vi "ESC controller 180319.vi"() -> ()   [LabVIEW 2022 SP3]
uses:
  <vilib>/Instr/_visa.llb/VISA Configure Serial Port (Instr).vi
panel:
  in  "OK Button":bool
  in  "Motor Capacity %":dbl(slide) scale=0.0..100.0
  in  "VISA resource name":refnum<visa-resource-name>="COM37"
  in  "exit":bool
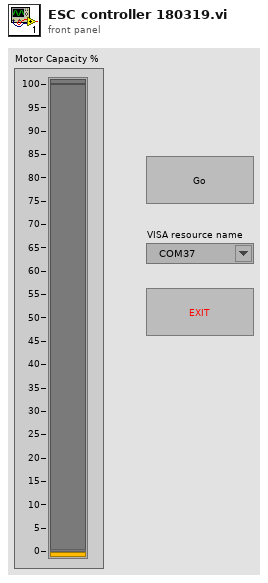
[diagram p1: front panel]
types:
  T1 = cluster{"baud rate":u32, "data bits":u16, "parity":enum16{"None", "Odd", "Even", "Mark", "Space"}, "stop bits":u16, "flow control":u16}
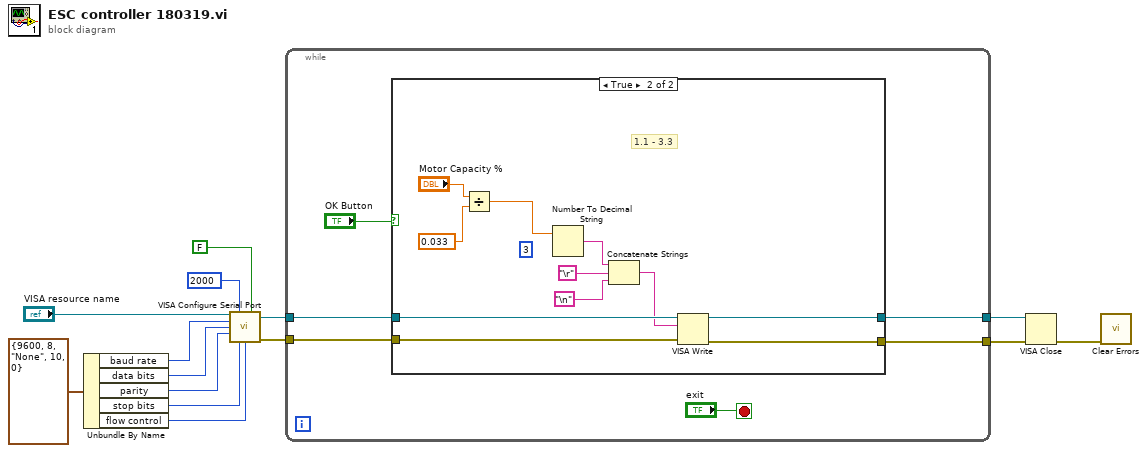
[diagram p0: block diagram]
diagram:
  n1 = Unbundle By Name(T1 {"baud rate"=9600, "data bits"=8, "parity"=enum."None", "stop bits"=10, "flow control"=0} ("Serial Settings")) -> ("baud rate"=w13:u32, "data bits"=w12:u16, "parity"=w11:enum16{"None", "Odd", "Even", "Mark", "Space"}, "stop bits"=w10:u16, "flow control"=w9:u16)
  n2 = call-poly "VISA Configure Serial Port"("VISA resource name"="VISA resource name", "timeout (10sec)"=u32 2000, "Enable Termination\nChar (T)"=FALSE ("Enable Termination\nChar (T)"), "baud rate (9600)"=w13, "data bits (8)"=w12, "parity (0:none)"=w11, "stop bits (10: 1 bit)"=w10, "flow control (0:none)"=w9) -> ("VISA resource name out"=w4:refnum<visa-resource-name>, "error out"=w5:errorcluster)  [unwired: 1 in, 5 out]
  n3 = while {
    tunnel: w5 -> [w20]
    tunnel: [w17] -> w3
    tunnel: [w16] -> w2
    tunnel: w4 -> [w19]
    stop <- "exit" stop-if-true
    n4 = case shown="True" "OK Button" {
      tunnel: w20 -> [w21 w33]
      tunnel: w19 -> [w22 w32]
      tunnel: [w21 w31] -> w17
      tunnel: [w22 w30] -> w16
      frame False {
      }
      frame True {
        (unwired) i16 3 ("width (-)")
        # "1.1 - 3.3"
        n5 = Divide(x="Motor Capacity %", y=0.033 ("x")) -> (x/y=w23:dbl)
        n6 = Number To Decimal String(number=w23) -> (decimal integer string=w26:string)  [unwired: 1 in]
        n7 = Concatenate Strings(w26, "\r", "\n") -> (w27:string)
        n8 = VISA Write(VISA resource name=w32, write buffer=w27, error in (no error)=w33) -> (VISA resource name out=w30:refnum<visa-resource-name>, error out=w31:errorcluster)  [unwired: 1 out]
      }
    }
  }
  n9 = VISA Close(VISA resource name=w2, error in (no error)=w3) -> (error out=w1:errorcluster)
  n10 = call <vilib>:"Clear Errors.vi"("error in (no error)"=w1) -> ()  [unwired: 5 in, 2 out]
